vi "TS.PropertyObject.GetSubpropertiesRecursive.vi"(8 "error in (no error)":errorcluster, 10 "parent property name":string, 11 "PropertyObject ref in":refnum<k7>) -> (0 "error out":errorcluster, 2 "subelements":T1(array[cluster]))   [LabVIEW 2019, in "Tools.lvlib"]
uses:
  Tools.lvlib
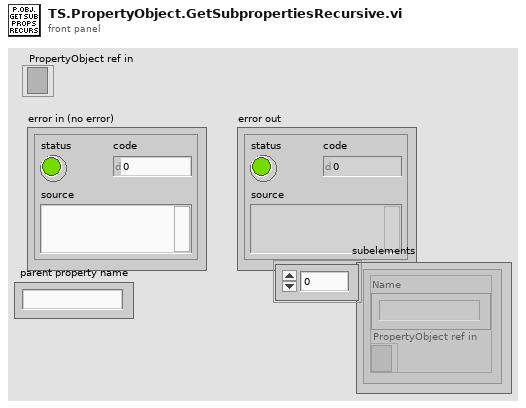
[diagram p1: front panel]
types:
  T1 = cluster{"Name":string, "PropertyObject ref in":refnum<k7>}[]
  T2 = cluster{"Name":string, "PropertyObject ref in":refnum<k7>}
  T3 = cluster{string, "PropertyObject ref in":refnum<k7>}
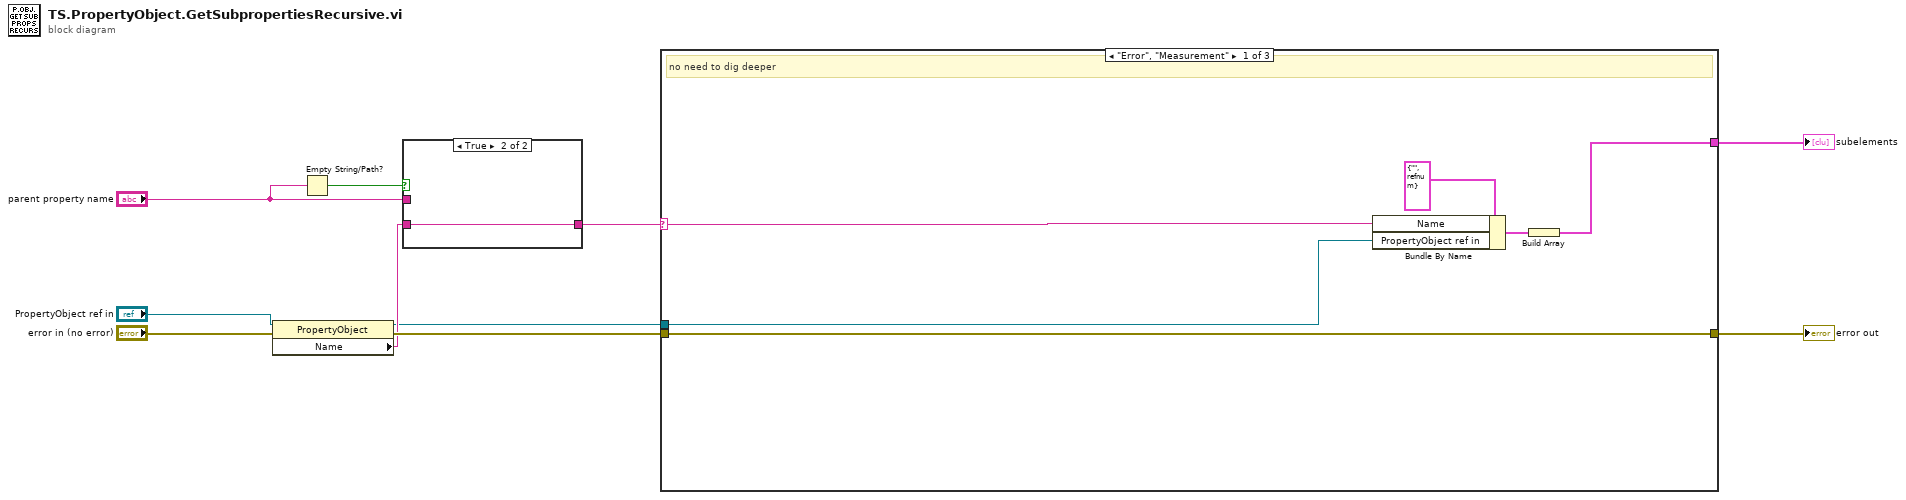
[diagram p0: block diagram]
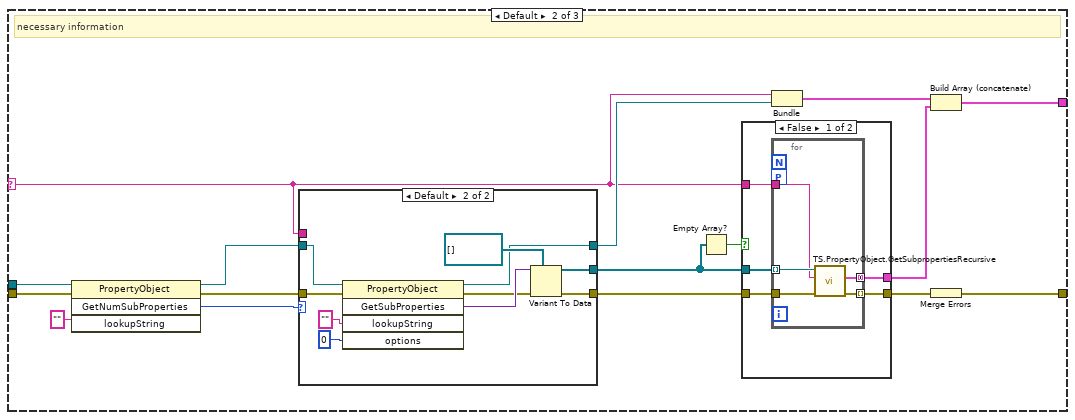
[diagram p2: hidden frame]
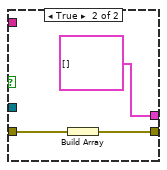
[diagram p3: hidden frame]
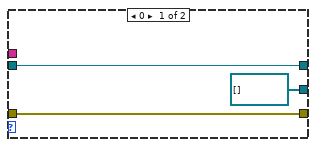
[diagram p4: hidden frame]
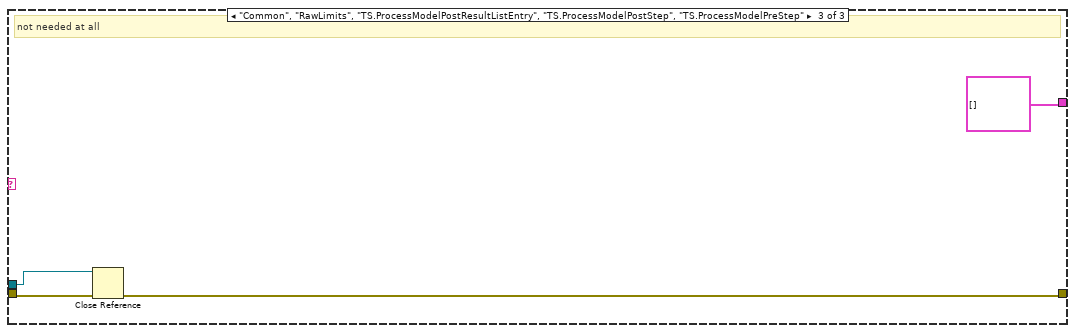
[diagram p5: hidden frame]
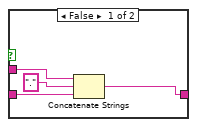
[diagram p6: hidden frame]
diagram:
  n1 = property class="PropertyObject"(reference="PropertyObject ref in", error in="error in (no error)") -> (reference out=w1:refnum<k7>, error out=w9:errorcluster, "Name"=w5:string)
  n2 = Empty String/Path?(string/path="parent property name") -> (empty?=w8:bool)
  n3 = case shown="True" w8 {
    tunnel: w5 -> [w12 w15]
    tunnel: [w11 w15] -> w2
    tunnel: "parent property name" -> [w14 _]
    frame False {
      n4 = Concatenate Strings(w14, "." ("string"), w12) -> (w11:string)
    }
    frame True {
    }
  }
  n5 = case shown="\"Error\", \"Measurement\"" w2 {
    selector: w2 -> [w19 w22 _]
    tunnel: w1 -> [w16 w35 w66]
    tunnel: w9 -> [w21 w34 w67]
    tunnel: [w17 w33 T1 []] -> w6
    tunnel: [w21 w25 w65] -> w4
    frame "Error", "Measurement" {
      # "no need to dig deeper"
      n6 = Bundle By Name(cluster=T2 {"Name"="", "PropertyObject ref in"=refnum}, "Name"=w19, "PropertyObject ref in"=w16) -> (w18:T2)
      n7 = Build Array(w18) -> (w17:T1)
    }
    frame Default {
      # "necessary information"
      n8 = invoke class="PropertyObject" method="GetNumSubProperties"(reference=w35, error in=w34, "lookupString"="") -> (reference out=w36:refnum<k7>, error out=w23:errorcluster, "GetNumSubProperties"=w37:i32)  [unwired: 1 in, 1 out]
      n9 = case shown="Default" w37 {
        tunnel: [w53 w58] -> w24
        tunnel: w36 -> [w51 w57]
        tunnel: w23 -> [w53 w56]
        tunnel: [refnum<k7>[] [] w55] -> w26
        tunnel: [w51 w54] -> w29
        tunnel: w22 -> [_ _]
        frame 0 {
        }
        frame Default {
          n10 = invoke class="PropertyObject" method="GetSubProperties"(reference=w57, error in=w56, "lookupString"="", "options"=0) -> (reference out=w54:refnum<k7>, error out=w59:errorcluster, "GetSubProperties"=w61:variant)  [unwired: 1 in, 2 out]
          n11 = Variant To Data(error in=w59, type=refnum<k7>[] [], Variant=w61) -> (data=w55:refnum<k7>[], error out=w58:errorcluster)
        }
      }
      n12 = Empty Array?(array=w26) -> (empty?=w27:bool)
      n13 = case shown="False" w27 {
        tunnel: [w42 T1 [] ("subelements")] -> w32
        tunnel: [w41 w48] -> w31
        tunnel: w22 -> [w40 _]
        tunnel: w26 -> [w39 _]
        tunnel: w24 -> [w38 w50]
        frame False {
          n14 = for {
            tunnel: w39 -> [w47] mode=indexing
            tunnel: w40 -> [w46]
            tunnel: w38 -> [w45]
            tunnel: [w44] -> w42 mode=concatenating
            tunnel: [w43] -> w41 mode=indexing
            workers-P: _ -> [_]
            n15 = call "TS.PropertyObject.GetSubpropertiesRecursive.vi"("error in (no error)"=w45, "parent property name"=w46, "PropertyObject ref in"=w47) -> ("error out"=w43:errorcluster, "subelements"=w44:T1)  [unwired: 7 in]
          }
        }
        frame True {
          n16 = Build Array(w50) -> (w48:errorcluster[])
        }
      }
      n17 = Bundle(w22, "PropertyObject ref in"=w29) -> (w28:T3)  [unwired: 1 in]
      n18 = Build Array (concatenate)(w28, w32) -> (w33:T1)
      n19 = Merge Errors(w31) -> (w25:errorcluster)
    }
    frame "Common", "RawLimits", "TS.ProcessModelPostResultListEntry", "TS.ProcessModelPostStep", "TS.ProcessModelPreStep" {
      # "not needed at all"
      n20 = Close Reference(reference=w66, error in (no error)=w67) -> (error out=w65:errorcluster)
    }
  }
  "error out" <- w4
  "subelements" <- w6
